vi "MainGUIRepository.vi"(0 "ReferenceIn":refnum<class "MasterGUI.lvclass">, 1 "Action(ReadRepository)":T1(ring), 5 "ErrorIn":errorcluster) -> (7 "QueueFromProcess":refnum<queue>, 9 "ProcessViRef":refnum<vi>, 10 "EventFromProcess":refnum<user-event>, 11 "ProcessSyncQueue":refnum<queue>, 14 "ReferenceOut":refnum<class "MasterGUI.lvclass">, 15 "EventsToProcess":refnum<user-event>, 17 "ProcessAlreadyStarted":bool, 19 "ErrorOut":errorcluster)   [LabVIEW 2021, in "MasterGUI.lvclass"]
uses:
  MasterGUI.lvclass
  MasterGUI.lvclass/MasterGUI.ctl
  MainGUI.ctl
  MainGUI.vi
panel:
  # "Use this indicator for sending messages to the Process VI"
  # "These indicators are used by the process VIs"
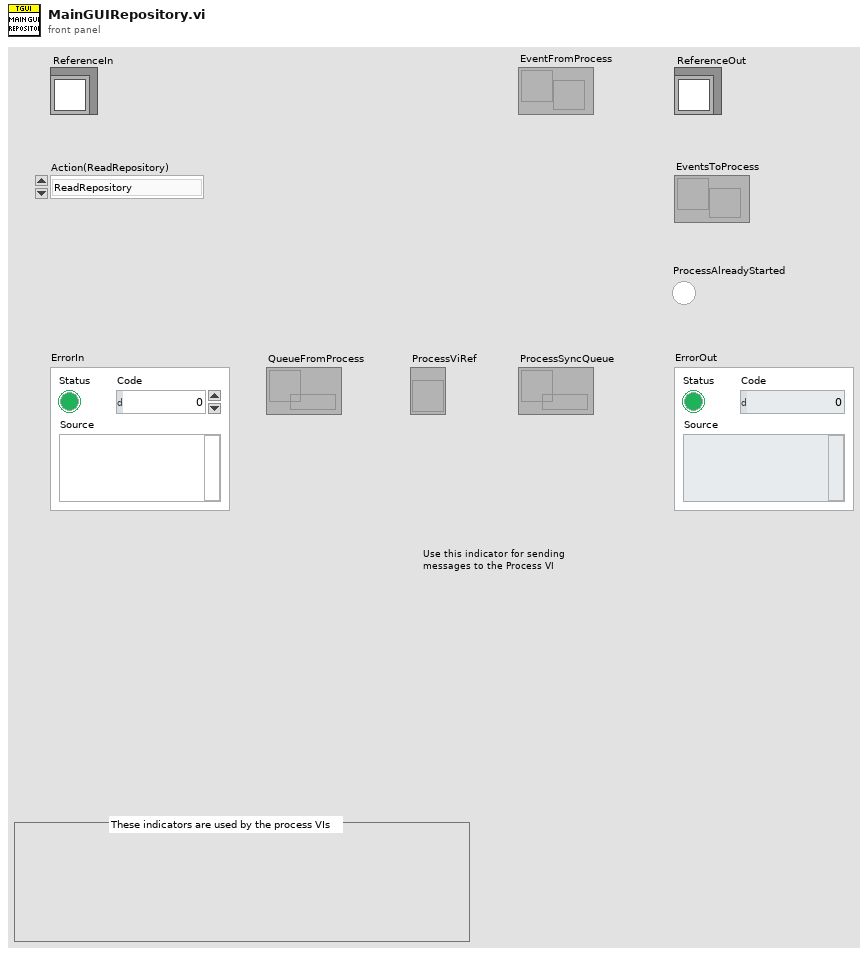
[diagram p1: front panel]
types:
  T1 = enum16{"ReadRepository", "CreateNew", "CreateOrLookUpExisting", "ReadRepositoryAndDestroy"}
  T2 = typedef "MasterGUI.lvclass/MainGUI.ctl" = cluster{"EventsToProcess":refnum<user-event>, "EventFromProcess":refnum<user-event>, "ProcessSyncQueue":refnum<queue>, "ProcessViRef":refnum<vi>, "QueueFromProcess":refnum<queue>}
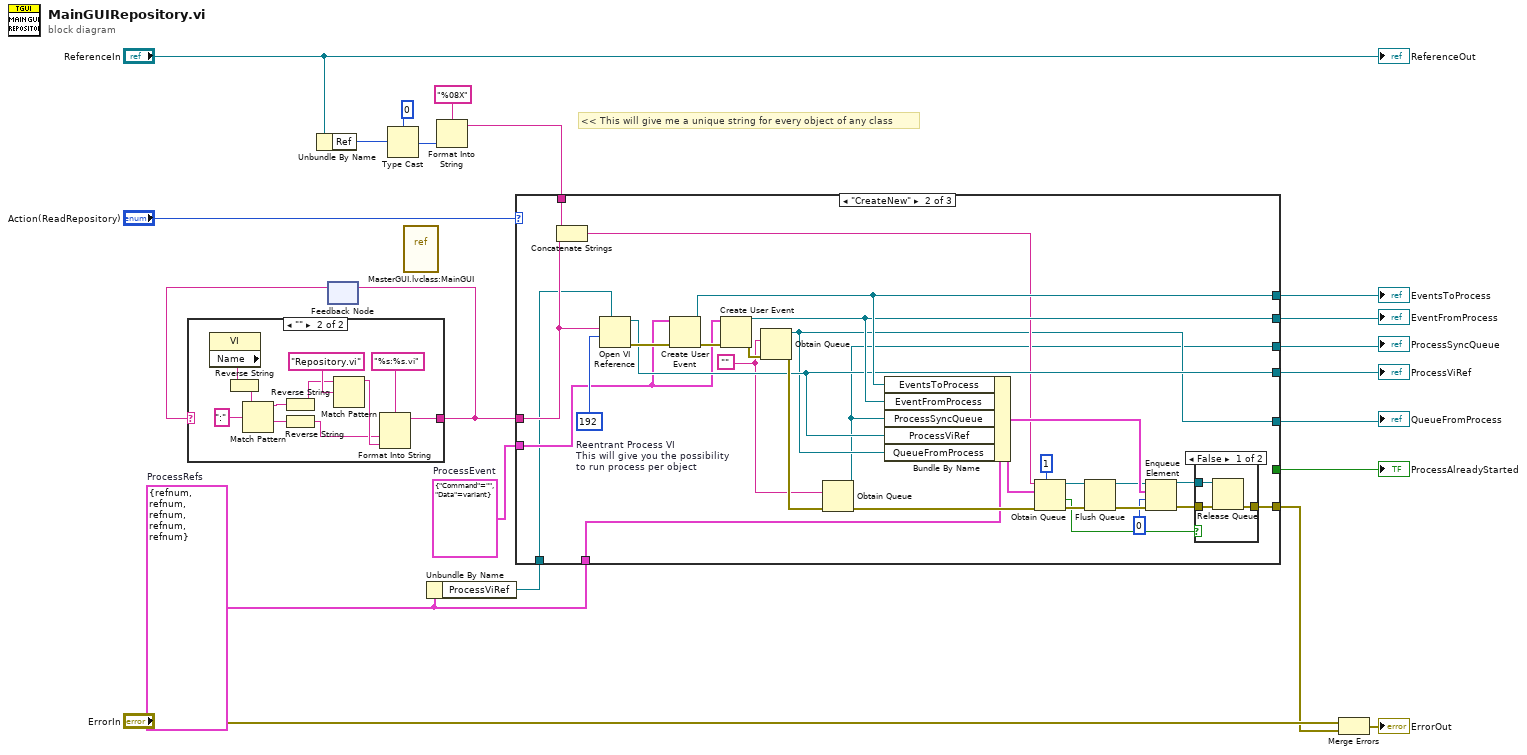
[diagram p0: block diagram]
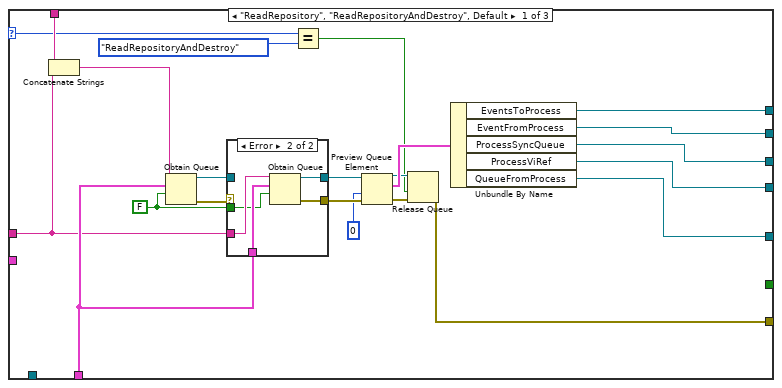
[diagram p3: hidden frame]
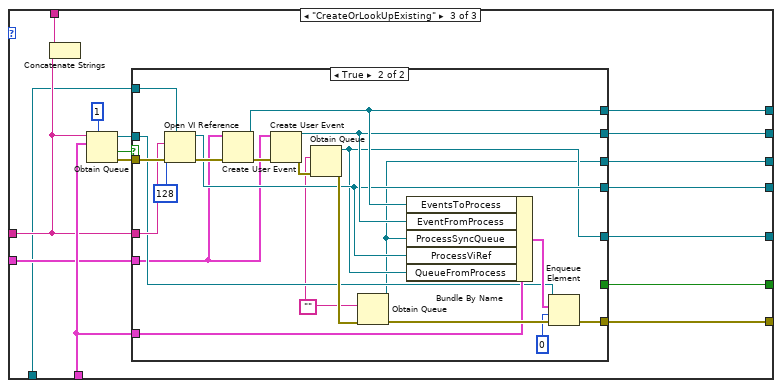
[diagram p6: hidden frame]
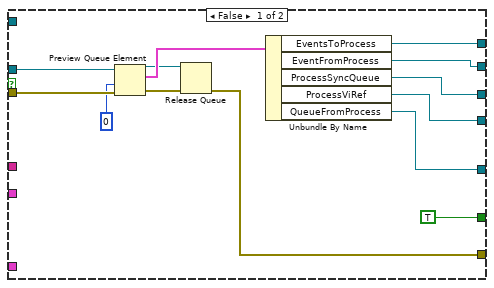
[diagram p7: hidden frame]
diagram:
  w1 = T2 {"EventsToProcess"=refnum, "EventFromProcess"=refnum, "ProcessSyncQueue"=refnum, "ProcessViRef"=refnum, "QueueFromProcess"=refnum}  # ProcessRefs
  w13 = cluster{"Command":string, "Data":variant} {"Command"="", "Data"=variant}  # ProcessEvent
  # "<< This will give me a unique string for every object of any class"
  n1 = Unbundle By Name("ReferenceIn") -> ("Ref"=w15:u32)
  n2 = feedback #1() -> (w11:string)  [unwired: 1 in]
  n3 = case shown="\"\"" w11 {
    selector: w11 -> [w22 _]
    tunnel: [w22 w23] -> w12
    frame Default {
    }
    frame "" {
      n4 = property class="VI"() -> ("Name"=w25:string)  [unwired: 2 in, 2 out]
      n5 = Reverse String(1:w25) -> (0:w26:string)
      n6 = Match Pattern(string=w26, regular expression=":") -> (before substring=w30:string, after substring=w27:string)  [unwired: 1 in, 2 out]
      n7 = Reverse String(1:w30) -> (0:w31:string)
      n8 = Reverse String(1:w27) -> (0:w29:string)
      n9 = Match Pattern(string=w31, regular expression="Repository.vi") -> (before substring=w33:string)  [unwired: 1 in, 3 out]
      n10 = Format Into String(format string="%s:%s.vi", w29, w33) -> (resulting string=w23:string)  [unwired: 2 in, 1 out]
    }
  }
  n11 = feedback-in #1(w12) -> ()
  n12 = Type Cast(type=u32 0, x=w15) -> (*(type *) &x=w18:u32)
  n13 = vi-ref "MasterGUI.lvclass:MainGUI.vi"() -> ()  [unwired: 1 out]
  n14 = Unbundle By Name(w1) -> ("ProcessViRef"=w10:refnum<vi>)
  n15 = Format Into String(format string="%08X", w18) -> (resulting string=w9:string)  [unwired: 2 in, 1 out]
  n16 = case shown="\"CreateNew\"" "Action(ReadRepository)" {
    selector: "Action(ReadRepository)" -> [w34 _ _]
    tunnel: [w47 w67 w107] -> w5
    tunnel: [w49 w82 w109] -> w7
    tunnel: [w48 w81 w108] -> w6
    tunnel: [w50 w80 w106] -> w4
    tunnel: w1 -> [w44 w74 w103]
    tunnel: w9 -> [w42 w73 w100]
    tunnel: [w52 w83 w111] -> w19
    tunnel: w12 -> [w41 w71 w97]
    tunnel: [_ _ w102] -> w2
    tunnel: w13 -> [_ w70 w99]
    tunnel: [w39 w69 w98] -> w3
    tunnel: w10 -> [_ w63 w96]
    frame "ReadRepository", "ReadRepositoryAndDestroy", Default {
      w43 = FALSE ("create if not found? (T)")
      n17 = Concatenate Strings(w42, w41) -> (w40:string)
      n18 = Obtain Queue(name (unnamed)=w40, element data type=w44, create if not found? (T)=w43) -> (queue out=w46:refnum<queue>, error out=w55:errorcluster)  [unwired: 2 in, 1 out]
      n19 = case shown="Error" w55 {
        selector: w55 -> [w57 _]
        tunnel: [w57 w62] -> w54
        tunnel: w46 -> [w56 _]
        tunnel: [w56 w59] -> w45
        tunnel: w44 -> [_ w61]
        tunnel: w41 -> [_ w60]
        tunnel: w43 -> [_ w58]
        frame No Error {
        }
        frame Error {
          n20 = Obtain Queue(name (unnamed)=w60, element data type=w61, create if not found? (T)=w58) -> (queue out=w59:refnum<queue>, error out=w62:errorcluster)  [unwired: 2 in, 1 out]
        }
      }
      n21 = Equal?(x=w34, y=T1."ReadRepositoryAndDestroy") -> (x = y?=w35:bool)
      n22 = Preview Queue Element(queue=w45, timeout in ms (-1)=0, error in (no error)=w54) -> (queue out=w37:refnum<queue>, element=w38:T2, error out=w53:errorcluster)  [unwired: 1 out]
      n23 = Release Queue(queue=w37, force destroy? (F)=w35, error in (no error)=w53) -> (error out=w52:errorcluster)  [unwired: 2 out]
      n24 = Unbundle By Name(w38) -> ("EventsToProcess"=w49:refnum<user-event>, "EventFromProcess"=w48:refnum<user-event>, "ProcessSyncQueue"=w47:refnum<queue>, "ProcessViRef"=w50:refnum<vi>, "QueueFromProcess"=w39:refnum<queue>)
    }
    frame "CreateNew" {
      w68 = ""
      w79 = 192  # Reentrant Process VI This will give you the possibility to run process per object
      n25 = Concatenate Strings(w73, w71) -> (w72:string)
      n26 = Open VI Reference(type specifier VI Refnum (for type only)=w63, vi path=w71, options=w79) -> (vi reference=w80:refnum<vi>, error out=w90:errorcluster)  [unwired: 3 in]
      n27 = Create User Event(user event datatype=w70, error in=w90) -> (user event=w82:refnum<user-event>, error out=w91:errorcluster)
      n28 = Create User Event(user event datatype=w70, error in=w91) -> (user event=w81:refnum<user-event>, error out=w89:errorcluster)
      n29 = Obtain Queue(element data type=w68, error in (no error)=w89) -> (queue out=w69:refnum<queue>, error out=w88:errorcluster)  [unwired: 3 in, 1 out]
      n30 = Obtain Queue(element data type=w68, error in (no error)=w88) -> (queue out=w67:refnum<queue>, error out=w87:errorcluster)  [unwired: 3 in, 1 out]
      n31 = Bundle By Name(cluster=w74, "EventsToProcess"=w82, "EventFromProcess"=w81, "ProcessSyncQueue"=w67, "ProcessViRef"=w80, "QueueFromProcess"=w69) -> (w77:T2)
      n32 = Obtain Queue(max queue size (-1, unlimited)=1, name (unnamed)=w72, element data type=w77, error in (no error)=w87) -> (queue out=w78:refnum<queue>, created new?=w65:bool, error out=w86:errorcluster)  [unwired: 1 in]
      n33 = Flush Queue(queue=w78, error in (no error)=w86) -> (queue out=w66:refnum<queue>, error out=w85:errorcluster)  [unwired: 1 out]
      n34 = Enqueue Element(queue=w66, element=w77, timeout in ms (-1)=0, error in (no error)=w85) -> (queue out=w64:refnum<queue>, error out=w84:errorcluster)  [unwired: 1 out]
      n35 = case shown="False" w65 {
        tunnel: w84 -> [w94 w95]
        tunnel: w64 -> [w92 _]
        tunnel: [w93 w95] -> w83
        frame False {
          n36 = Release Queue(queue=w92, error in (no error)=w94) -> (error out=w93:errorcluster)  [unwired: 1 in, 2 out]
        }
        frame True {
        }
      }
    }
    frame "CreateOrLookUpExisting" {
      n37 = Concatenate Strings(w100, w97) -> ()  [unwired: 1 out]
      n38 = Obtain Queue(max queue size (-1, unlimited)=1, name (unnamed)=w97, element data type=w103) -> (queue out=w104:refnum<queue>, created new?=w105:bool, error out=w110:errorcluster)  [unwired: 2 in]
      n39 = case shown="True" w105 {
        tunnel: [w121 w138] -> w109
        tunnel: [w120 w137] -> w108
        tunnel: [w119 w127] -> w107
        tunnel: [w118 w136] -> w106
        tunnel: [w122 w145] -> w111
        tunnel: w103 -> [_ w135]
        tunnel: w110 -> [w124 w142]
        tunnel: w97 -> [_ w132]
        tunnel: w104 -> [w116 w131]
        tunnel: [TRUE _] -> w102
        tunnel: w99 -> [_ w130]
        tunnel: [w113 w129] -> w98
        tunnel: w96 -> [_ w126]
        frame False {
          n40 = Preview Queue Element(queue=w116, timeout in ms (-1)=0, error in (no error)=w124) -> (queue out=w112:refnum<queue>, element=w115:T2, error out=w123:errorcluster)  [unwired: 1 out]
          n41 = Release Queue(queue=w112, error in (no error)=w123) -> (error out=w122:errorcluster)  [unwired: 1 in, 2 out]
          n42 = Unbundle By Name(w115) -> ("EventsToProcess"=w121:refnum<user-event>, "EventFromProcess"=w120:refnum<user-event>, "ProcessSyncQueue"=w119:refnum<queue>, "ProcessViRef"=w118:refnum<vi>, "QueueFromProcess"=w113:refnum<queue>)
        }
        frame True {
          w128 = ""
          n43 = Open VI Reference(type specifier VI Refnum (for type only)=w126, vi path=w132, options=128, error in (no error)=w142) -> (vi reference=w136:refnum<vi>, error out=w143:errorcluster)  [unwired: 2 in]
          n44 = Create User Event(user event datatype=w130, error in=w143) -> (user event=w138:refnum<user-event>, error out=w144:errorcluster)
          n45 = Create User Event(user event datatype=w130, error in=w144) -> (user event=w137:refnum<user-event>, error out=w141:errorcluster)
          n46 = Obtain Queue(element data type=w128, error in (no error)=w141) -> (queue out=w129:refnum<queue>, error out=w140:errorcluster)  [unwired: 3 in, 1 out]
          n47 = Obtain Queue(element data type=w128, error in (no error)=w140) -> (queue out=w127:refnum<queue>, error out=w139:errorcluster)  [unwired: 3 in, 1 out]
          n48 = Bundle By Name(cluster=w135, "EventsToProcess"=w138, "EventFromProcess"=w137, "ProcessSyncQueue"=w127, "ProcessViRef"=w136, "QueueFromProcess"=w129) -> (w134:T2)
          n49 = Enqueue Element(queue=w131, element=w134, timeout in ms (-1)=0, error in (no error)=w139) -> (error out=w145:errorcluster)  [unwired: 2 out]
        }
      }
    }
  }
  "ProcessSyncQueue" <- w5
  "EventsToProcess" <- w7
  "EventFromProcess" <- w6
  "ProcessViRef" <- w4
  "ProcessAlreadyStarted" <- w2
  "QueueFromProcess" <- w3
  n50 = Merge Errors("ErrorIn", w19) -> (→"ErrorOut":errorcluster)
  "ReferenceOut" <- "ReferenceIn"
